vi "LAB1.vi"() -> ()   [LabVIEW 2025]
panel:
  out "Tank":dbl(slide) scale=0.0..10.0
  in  "Slide":dbl(slide) scale=0.0..10.0
  out "Thermometer":dbl(slide) scale=0.0..100.0
  in  "Knob":dbl(knob) scale=0.0..10.0
  in  "Numeric":dbl
  out "Boolean 5":bool
  in  "Boolean 4":bool
  in  "Boolean 3":bool
  in  "stop":bool
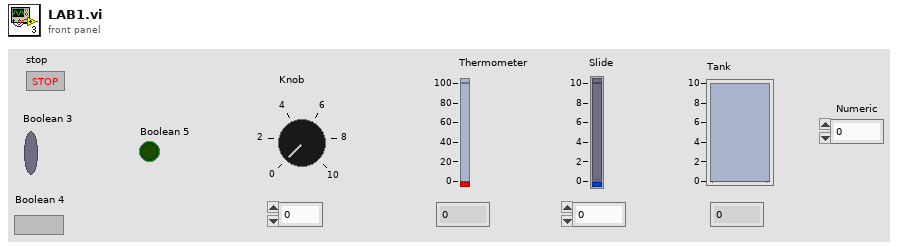
[diagram p1: front panel]
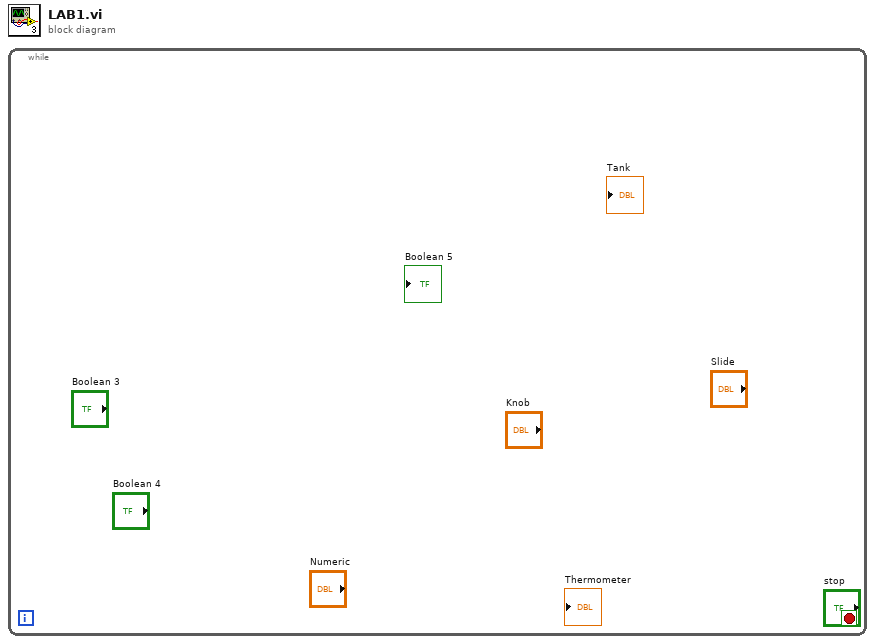
[diagram p0: block diagram]
diagram:
  n1 = while {
    stop <- _ stop-if-true
  }
